vi "sync and trig.vi"(8 "error in (no error)":errorcluster, 10 "time calibrate":dbl[](array[numeric]), 11 "5785_2_x_1600MHz in":refnum<class "5785_2_x_1600MHz.lvclass">) -> (0 "error out":errorcluster, 3 "5785_2_x_1600MHz out":refnum<class "5785_2_x_1600MHz.lvclass">)   [LabVIEW 2021, in "5785_2_x_1600MHz.lvclass"]
uses:
  5785_2_x_1600MHz.lvclass
  5785_2_x_1600MHz.lvclass/5785_2_x_1600MHz.ctl
  <vilib>/Utility/error.llb/Error Cluster From Error Code.vi
  <vilib>/rvi/errors/niLvFpgaAdjustHostInterfaceError.vi
  <instrlib>/_niInstr/Streaming/v1/Host/Public/Start Continuous Stream.vi
  <vilib>/rvi/interface/nirviReadWriteControl/nirviReadWriteControl.xnode
  <instrlib>/_niInstr/Streaming/v1/Host/niInstr Streaming v1 Host.lvlib
  <resource>/objmgr/sessionReference.rc
  NiFpgaLv.dll
  <vilib>/rvi/interface/Simulation/niFpgaSimulationCallBeginRW.vi
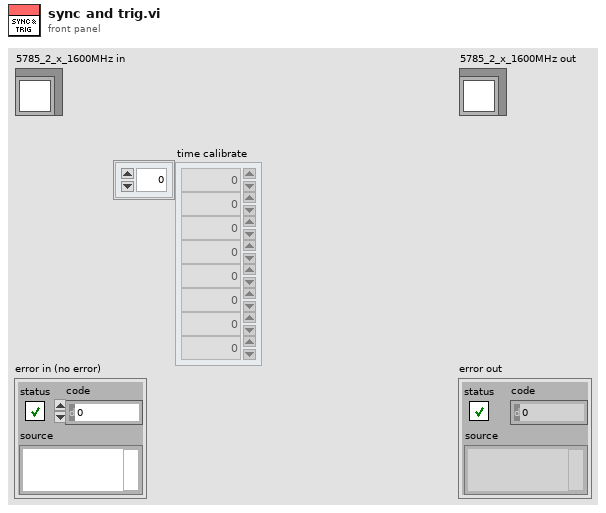
[diagram p1: front panel]
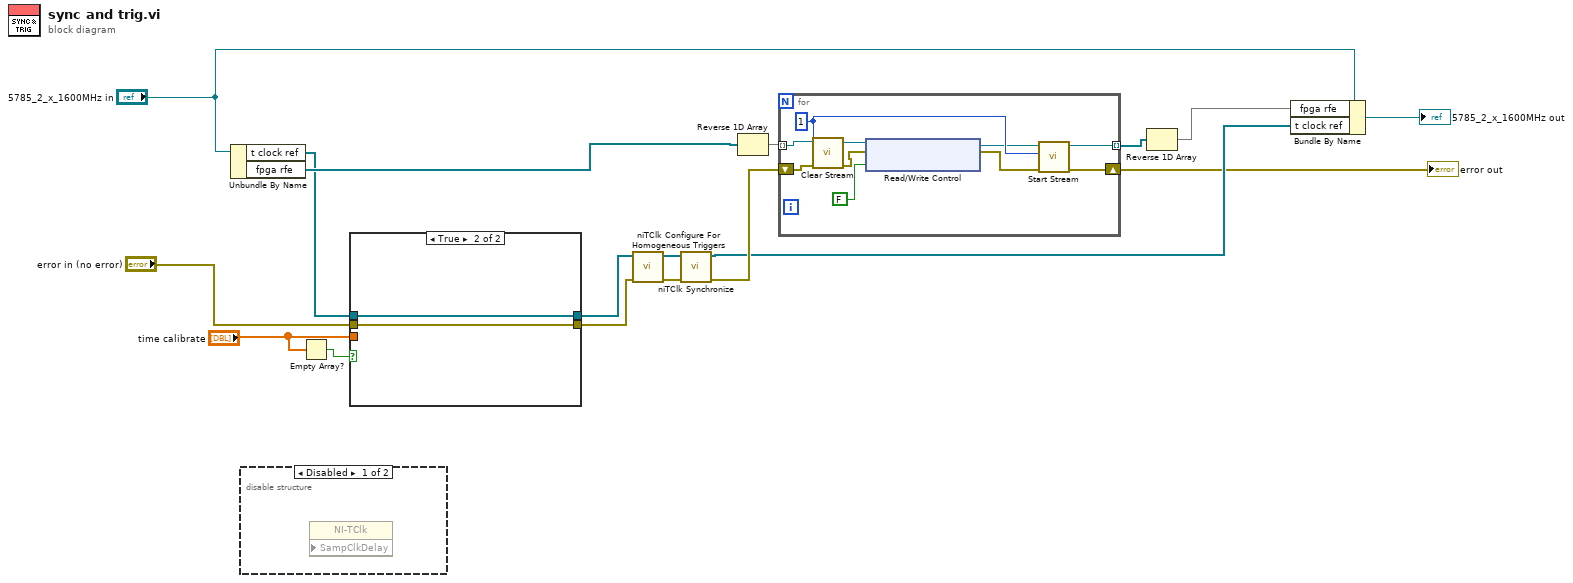
[diagram p0: block diagram]
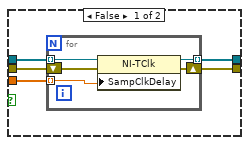
[diagram p2: hidden frame]
diagram:
  n1 = Unbundle By Name("5785_2_x_1600MHz in") -> ("t clock ref"=w5:refnum<k20>[], "fpga rfe"=w7:refnum<k20>[])
  n2 = disable-structure shown="Disabled" {
    frame Disabled {
      n3 = property class="NI-TClk" props=["SampClkDelay"]() -> ()  [unwired: 3 in, 2 out]
    }
    frame Enabled {
    }
  }
  n4 = Empty Array?(array="time calibrate") -> (empty?=w1:bool)
  n5 = case shown="True" w1 {
    tunnel: "error in (no error)" -> [w22 w28]
    tunnel: [w21 w28] -> w8
    tunnel: [w20 w29] -> w6
    tunnel: w5 -> [w19 w29]
    tunnel: "time calibrate" -> [w18 _]
    frame False {
      n6 = for {
        tunnel: w19 -> [w27] mode=indexing
        tunnel: [w26] -> w20 mode=indexing
        shift-right: [w24] -> w21
        shift-left: w22 -> [w25]
        tunnel: w18 -> [w23] mode=indexing
        n7 = property class="NI-TClk"(reference=w27, error in=w25, "SampClkDelay"=w23) -> (reference out=w26:refnum<k20>, error out=w24:errorcluster)
      }
    }
    frame True {
    }
  }
  n8 = call <instrlib>:"niTClk Configure For Homogeneous Triggers.vi"("error in (no error)"=w8, "sessions"=w6) -> ("error out"=w14:errorcluster, "sessions out"=w15:refnum<k20>[])  [unwired: 8 in]
  n9 = call <instrlib>:"niTClk Synchronize.vi"("error in (no error)"=w14, "sessions"=w15) -> ("error out"=w17:errorcluster, "sessions out"=w13:refnum<k20>[])  [unwired: 8 in]
  n10 = Reverse 1D Array(array=w7) -> (reversed array=w16:refnum<k20>[])
  n11 = for {
    tunnel: w16 -> [w35] mode=indexing
    shift-right: [w38] -> w11
    shift-left: w17 -> [w34]
    tunnel: [w37] -> w4 mode=indexing
    w39 = 1 ("stream index")
    n12 = call <instrlib>:"Clear Stream.vi"("error in (no error)"=w34, "stream index"=w39, "refnum in"=w35) -> ("error out"=w33:errorcluster, "refnum out"=w32:refnum<k20>)  [unwired: 7 in]
    n13 = xnode "Read/Write Control"("FPGA VI Reference In"=w32, "error in"=w33, "reset system clock"=FALSE) -> ("FPGA VI Reference Out"=w30:refnum<k20>, "error out"=w31:errorcluster)
    n14 = call-poly <instrlib>:"Start Stream.vi"("error in (no error)"=w31, "stream index"=w39, "refnum in"=w30) -> ("error out"=w38:errorcluster, "refnum out"=w37:refnum<k20>)  [unwired: 7 in]
  }
  "error out" <- w11
  n15 = Reverse 1D Array(array=w4) -> (reversed array=w3:refnum<k20>[])
  n16 = Bundle By Name(cluster="5785_2_x_1600MHz in", "fpga rfe"=w3, "t clock ref"=w13) -> (→"5785_2_x_1600MHz out":refnum<class "5785_2_x_1600MHz.lvclass">)
